vi "Configure Channel Core.vi"(0 "IVI_Scope in":refnum<class "IVI_Scope.lvclass">, 1 "channel enabled (True)":bool=TRUE, 2 "channel name (\"CHANNEL1\")":string="CHANNEL1", 3 "probe attenuation (1:1.0)":dbl=1.0 format="%.3f", 4 "vertical offset (0.0 V)":dbl[unit] format="%.3f", 5 "error in (no error)":errorcluster, 6 "vertical coupling (DC)":i32(ring)=1 items=["AC", "DC", "GND"], 8 "vertical range (10.0 V)":dbl[unit]=10.0 format="%.3f") -> (14 "IVI_Scope out":refnum<class "IVI_Scope.lvclass">, 19 "error out":errorcluster)   [LabVIEW 2013, in "IVI_Scope.lvlib" / "IVI_Scope.lvclass"]
doc: "This VI configures the most commonly configured properties of the oscilloscope channel sub-system. These properties are the range, offset, coupling, probe attenuation, and whether the channel is enabled."
uses:
  IVI_Scope.lvclass
  IVI_Scope.lvclass/IVI_Scope.ctl
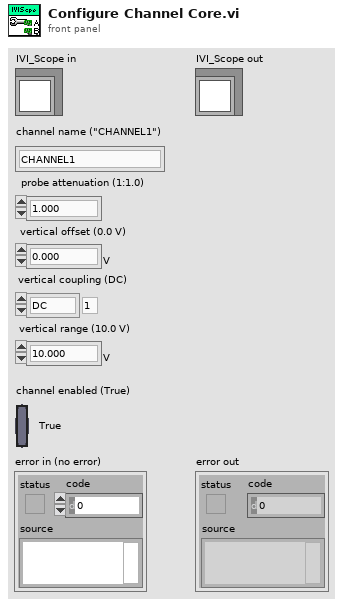
[diagram p1: front panel]
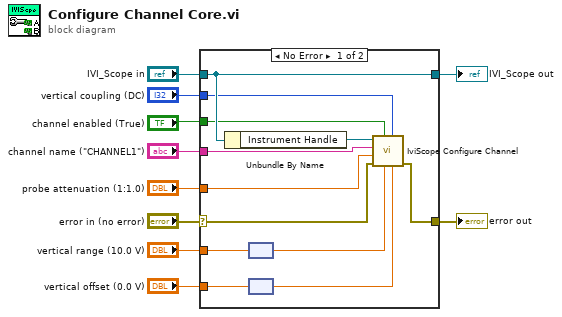
[diagram p0: block diagram]
diagram:
  n1 = case shown="No Error" "error in (no error)" {
    selector: "error in (no error)" -> [w18 w24]
    tunnel: [w17 w24] -> w9
    tunnel: [w22 w23] -> w7
    tunnel: "IVI_Scope in" -> [w22 w23]
    tunnel: "channel name (\"CHANNEL1\")" -> [w20 _]
    tunnel: "probe attenuation (1:1.0)" -> [w19 _]
    tunnel: "vertical range (10.0 V)" -> [w16 _]
    tunnel: "vertical offset (0.0 V)" -> [w15 _]
    tunnel: "channel enabled (True)" -> [w14 _]
    tunnel: "vertical coupling (DC)" -> [w13 _]
    frame No Error {
      n2 = Unbundle By Name(w22) -> ("Instrument Handle"=w21:refnum<k15>)
      n3 = node(w16) -> (w12:dbl)
      n4 = node(w15) -> (w11:dbl)
      n5 = call <vilib>:"IviScope Configure Channel.vi"("vertical offset (0.0 V)"=w11, "vertical coupling (DC)"=w13, "vertical range (10.0 V)"=w12, "channel enabled (True)"=w14, "error in (no error)"=w18, "probe attenuation (1:1.0)"=w19, "channel name (\"CHANNEL1\")"=w20, "instrument handle"=w21) -> ("error out"=w17:errorcluster)  [unwired: 2 in, 1 out]
    }
    frame Error {
    }
  }
  "error out" <- w9
  "IVI_Scope out" <- w7
